vi "Elevator Logic Test.vi"() -> ()   [LabVIEW 2014]
uses:
  <vilib>/addons/control/pid/NI_PID_pid.lvlib
  <vilib>/addons/control/pid/pid.llb/PID Output Rate Limiter (DBL).vi
  Common Code/Elevator State.ctl
  Robot Code/Elevator/Elevator Command.ctl
panel:
  in  "Command":T1
  in  "Presets":T2
  out "Tote Count":dbl
  out "Has Trashcan":bool
  out "State":T3
  in  "Trashcan Sensor":bool
  in  "Sim speed":dbl=1.0 format="%.2f"
  in  "High IR":bool
  in  "Low IR":bool
  out "Ejector Piston":bool
  out "Level":dbl(slide) scale=0.0..10.0
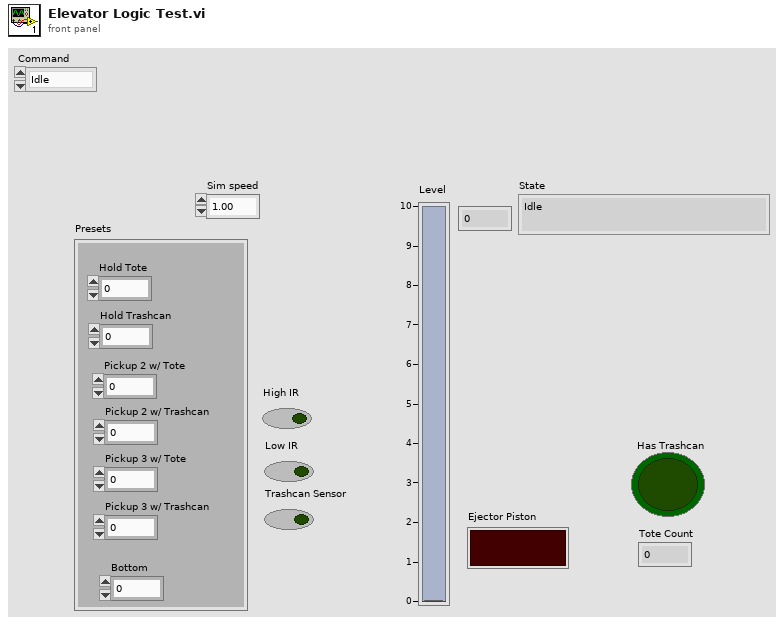
[diagram p1: front panel]
types:
  T1 = typedef "Elevator Command.ctl" = enum16{"Idle", "Load 1", "Load 2", "Load 3", "Drop Stack", "Eject Stack", "Load Trashcan"}
  T2 = cluster{"Hold Tote":dbl, "Hold Trashcan":dbl, "Pickup 2 w/ Tote":dbl, "Pickup 2 w/ Trashcan":dbl, "Pickup 3 w/ Tote":dbl, "Pickup 3 w/ Trashcan":dbl, "Bottom":dbl}
  T3 = typedef "Elevator State.ctl" = enum16{"Idle", "Goto Load Position", "Wait for Load", "Load Drop", "Load Lift", "Drop Stack"}
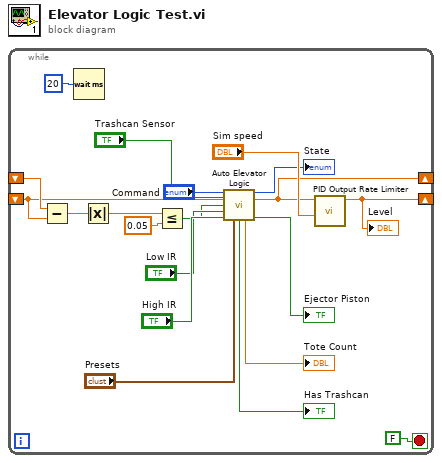
[diagram p0: block diagram]
diagram:
  n1 = while {
    shift-right: [w13] -> _
    shift-left: _ -> [w10]
    shift-right: [w12] -> _
    shift-left: _ -> [w11]
    stop <- FALSE stop-if-true
    n2 = Subtract(x=w11, y=w10) -> (x-y=w9:dbl)
    n3 = Wait (ms)(milliseconds to wait=u32 20) -> ()  [unwired: 1 out]
    n4 = Absolute Value(x=w9) -> (abs(x)=w8:dbl)
    n5 = Less Or Equal?(x=w8, y=0.05) -> (x <= y?=w6:bool)
    n6 = call "Auto Elevator Logic.vi"("Command"="Command", 1:"Trashcan Sensor", 5:w10, "Elevator Sensors In"=w6, 9:"Low IR", 11:"High IR", "Presets"="Presets") -> ("State"=→"State":T3, "Position Out"=w12:dbl, "Add Trashcan"=→"Has Trashcan":bool, "Tote Count Delta"=→"Tote Count":dbl, "Ejector Piston"=→"Ejector Piston":bool)  [unwired: 2 in, 2 out]
    n7 = call-poly <vilib>:"PID Output Rate Limiter.vi"("output rate (EGU/min)"="Sim speed", "input (controller output)"=w12) -> ("output"=w13:dbl)  [unwired: 6 in, 1 out]
    "Level" <- w13
  }
